vi "求方程的根（牛顿迭代法）.vi"() -> ()   [LabVIEW 2012]
doc: "功能：\n\n利用牛顿迭代法求一个数的n次方根\n\n\ncsxcs_366创建"
panel:
  out "根":dbl
  in  "预设值":dbl
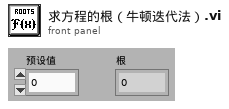
[diagram p1: front panel]
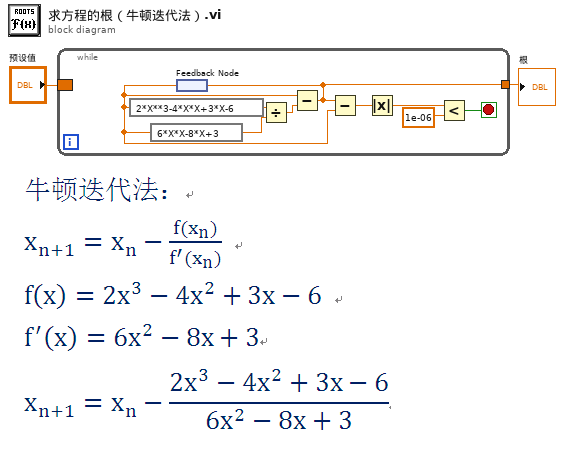
[diagram p0: block diagram]
diagram:
  n1 = while {
    border: "预设值" -> [_]
    tunnel: [w3] -> w1
    stop <- w8 stop-if-true
    n2 = feedback #1() -> (w4:dbl)
    n3 = expression code="2*X**3-4*X*X+3*X-6"(w4) -> (w7:dbl)
    n4 = expression code="6*X*X-8*X+3"(w4) -> (w6:dbl)
    n5 = Divide(x=w7, y=w6) -> (x/y=w5:dbl)
    n6 = Subtract(x=w4, y=w5) -> (x-y=w3:dbl)
    n7 = feedback-in #1(w3) -> ()
    n8 = Subtract(x=w3, y=w4) -> (x-y=w11:dbl)
    n9 = Absolute Value(x=w11) -> (abs(x)=w10:dbl)
    n10 = Less?(x=w10, y=1e-06) -> (x < y?=w8:bool)
  }
  "根" <- w1
